vi "classify error.vi"(8 "error to classify":errorcluster, 10 "attempt recovery?":bool, 11 "Modbus Slave runtime in":refnum<class "Modbus Slave runtime.lvclass">) -> (0 "classified error":errorcluster, 2 "error classification":T1, 3 "Modbus Slave runtime out":refnum<class "Modbus Slave runtime.lvclass">)   [LabVIEW 2013, in "Modbus Slave runtime.lvclass"]
doc: "Allows a module to classify an error generated at any point during execution. This <b>error classification</b> can then be used by calling code to determine if execution can continue. In addition, this function can be used to allow a component to clear an error, convert an error to a warning, or attempt to recover from an error. Recovery may be attempted only if <b>attempt recovery?</b> is true.Platypus Framework 1.0.1.65\nNI Systems Engineering - National Instruments"
uses:
  Modbus Slave runtime.lvclass
  <vilib>/NI/Tag Bus Module Framework/runtime/error classification.ctl
  <vilib>/NI/Tag Bus Module Framework/runtime/TBM module execution interface.lvclass
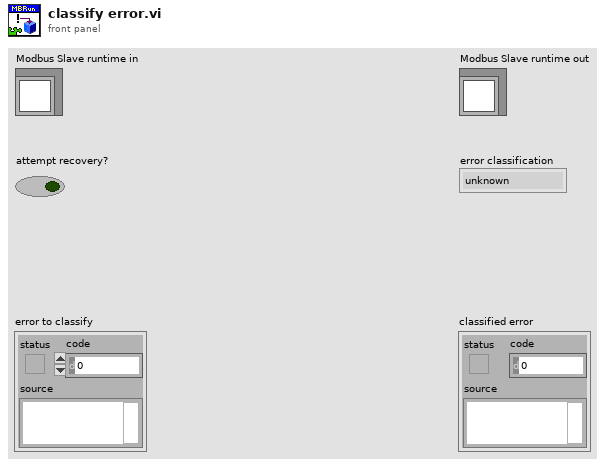
[diagram p1: front panel]
types:
  T1 = typedef "TBM module execution interface.lvclass/error classification.ctl" = enum16{"unknown", "none", "trivial", "recoverable", "critical"}
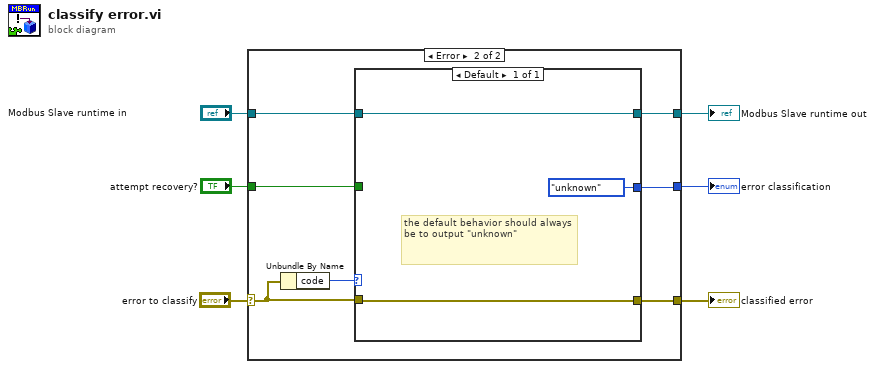
[diagram p0: block diagram]
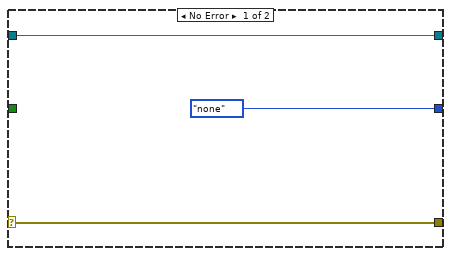
[diagram p2: hidden frame]
diagram:
  n1 = case shown="Error" "error to classify" {
    selector: "error to classify" -> [w8 w15]
    tunnel: "attempt recovery?" -> [_ w10]
    tunnel: [w9 w11] -> w4
    tunnel: "Modbus Slave runtime in" -> [w9 w12]
    tunnel: [w8 w14] -> w2
    tunnel: [error_classification."none" ("error classification") w13] -> w1
    frame No Error {
    }
    frame Error {
      n2 = Unbundle By Name(w15) -> ("code"=w16:i32)
      n3 = case shown="Default" w16 {
        tunnel: w15 -> [w17]
        tunnel: [w17] -> w14
        tunnel: [error_classification."unknown" ("error classification")] -> w13
        tunnel: w12 -> [w18]
        tunnel: [w18] -> w11
        tunnel: w10 -> [_]
        frame Default {
          # "the default behavior should always be to output \"unknown\""
        }
      }
    }
  }
  "Modbus Slave runtime out" <- w4
  "error classification" <- w1
  "classified error" <- w2
